vi "Begin.vi"(8 "error in (no error)":errorcluster, 11 "Trace Controller in":refnum<class "Trace Controller.lvclass">) -> (0 "error out":errorcluster, 3 "Trace Controller out":refnum<class "Trace Controller.lvclass">)   [LabVIEW 2014, in "Robot Actor Framework.lvlib" / "Trace.lvlib" / "Trace Controller.lvclass"]
uses:
  Trace Controller.lvclass
  Trace Controller.lvclass/Trace Controller.ctl
  Trace Class/Trace.lvclass
  System Actor/System Actor Class/System Actor.lvclass
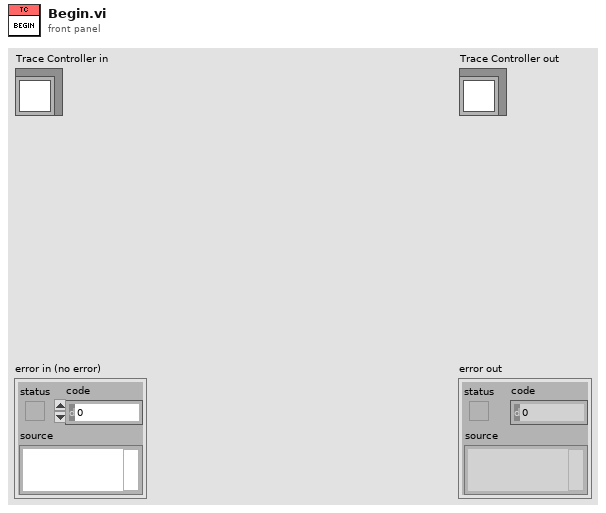
[diagram p1: front panel]
types:
  T1 = enum16{"Critical", "Error", "Warning", "Informational", "Debug"}
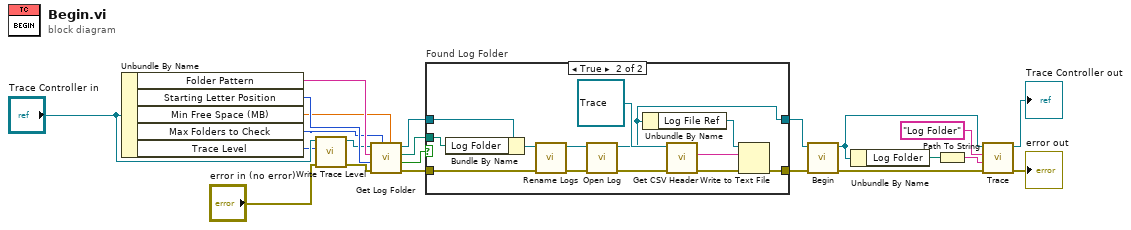
[diagram p0: block diagram]
diagram:
  n1 = Unbundle By Name("Trace Controller in") -> ("Folder Pattern"=w10:string, "Starting Letter Position"=w9:i32, "Min Free Space (MB)"=w8:dbl, "Max Folders to Check"=w7:u32, "Trace Level"=w3:T1)
  n2 = call-dynamic "Write Trace Level.vi"("error in (no error)"="error in (no error)", "Trace Level"=w3, "System Actor in"="Trace Controller in") -> ("error out"=w1:errorcluster, "System Actor out"=w4:refnum<class "Trace Controller.lvclass">)  [unwired: 7 in]
  n3 = call-dynamic "Get Log Folder.vi"("Min Free Space (MB)"=w8, "Max Folders to Check"=w7, "error in (no error)"=w1, "Starting Letter Position"=w9, "Folder Pattern"=w10, "Trace Controller in"=w4) -> ("error out"=w11:errorcluster, "Folder Found?"=w6:bool, "Folder"=w13:path, "Trace Controller out"=w12:refnum<class "Trace Controller.lvclass">)  [unwired: 2 in]
  n4 = case "Found Log Folder" shown="True" w6 {
    tunnel: [w24 w33] -> w22
    tunnel: [w23 w31] -> w21
    tunnel: w13 -> [_ w27]
    tunnel: w12 -> [w23 w26]
    tunnel: w11 -> [w24 w25]
    frame False {
    }
    frame True {
      n5 = Bundle By Name(cluster=w26, "Log Folder"=w27) -> (w37:refnum<class "Trace Controller.lvclass">)
      n6 = call-dynamic "Rename Logs.vi"("error in (no error)"=w25, "Trace Controller in"=w37) -> ("error out"=w34:errorcluster, "Trace Controller out"=w35:refnum<class "Trace Controller.lvclass">)  [unwired: 8 in]
      n7 = call-dynamic "Open Log.vi"("error in (no error)"=w34, "Trace Controller in"=w35) -> ("error out"=w29:errorcluster, "Trace Controller out"=w31:refnum<class "Trace Controller.lvclass">)  [unwired: 8 in]
      n8 = Unbundle By Name(w31) -> ("Log File Ref"=w30:refnum<file>)
      n9 = call-dynamic "Get CSV Header.vi"("error in (no error)"=w29, "Trace in"=refnum<class "Trace.lvclass"> refnum ("Robot Actor Framework.lvlib:Trace.lvlib:Trace.lvclass")) -> ("error out"=w28:errorcluster, "CSV Header"=w32:string)  [unwired: 7 in, 1 out]
      n10 = Write to Text File(file (use dialog)=w30, text=w32, error in=w28) -> (error out=w33:errorcluster)  [unwired: 1 in, 2 out]
    }
  }
  n11 = call-parent "Begin.vi"("error in (no error)"=w22, "System Actor in"=w21) -> ("error out"=w15:errorcluster, "System Actor out"=w19:refnum<class "Trace Controller.lvclass">)  [unwired: 8 in]
  n12 = Unbundle By Name(w19) -> ("Log Folder"=w18:path)
  n13 = Path To String(path=w18) -> (string=w17:string)
  n14 = call-dynamic "Trace.vi"("error in (no error)"=w15, "System Message"=w17, "System Action"="Log Folder", "System Actor in"=w19) -> ("error out"=→"error out":errorcluster, "System Actor out"=→"Trace Controller out":refnum<class "Trace Controller.lvclass">)  [unwired: 6 in]
